vi "tearDown.vi"(8 "error in (no error)":errorcluster, 11 "reference in":refnum<class "Interface Framework Multiple Objects.lvclass">) -> (0 "error out":errorcluster, 3 "reference out":refnum<class "Interface Framework Multiple Objects.lvclass">)   [LabVIEW 2009, in "Interface Framework Multiple Objects.lvclass"]
doc: "tearDown runs after the test method has completed. Use this method to clean up any operations or references that were opened by setUp or the test method. Unit tests should be independent of other unit tests so this VI should ensure that the next test can run in a 'clean' test environment."
uses:
  Interface Framework Multiple Objects.lvclass
  Numeric Test Object/Numeric Test Object.lvclass
  Interface Framework Multiple Objects.lvclass/Interface Framework Multiple Objects.ctl
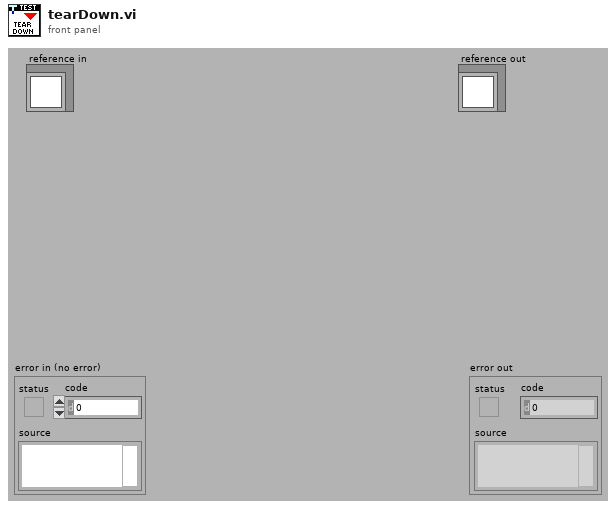
[diagram p1: front panel]
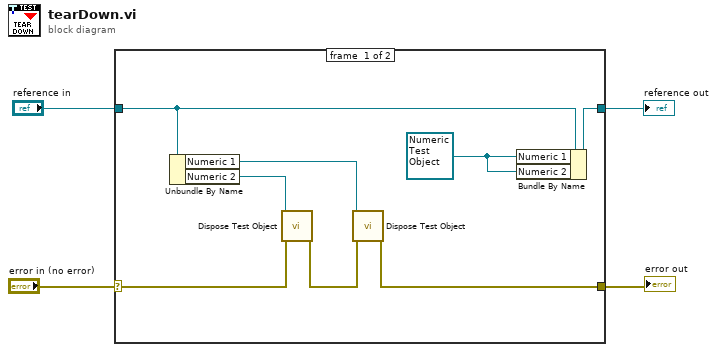
[diagram p0: block diagram]
diagram:
  n1 = case shown="No Error" "error in (no error)" {
    selector: "error in (no error)" -> [w11 w14]
    tunnel: [w9 w14] -> w3
    tunnel: [w6 w13] -> w1
    tunnel: "reference in" -> [w12 w13]
    frame #0 {
      w5 = refnum<class "Numeric Test Object.lvclass"> refnum ("Numeric 1")
      n2 = Unbundle By Name(w12) -> ("Numeric 1"=w7:refnum<class "Numeric Test Object.lvclass">, "Numeric 2"=w8:refnum<class "Numeric Test Object.lvclass">)
      n3 = call "Dispose Test Object.vi"("error in (no error)"=w11, "Numeric"=w8) -> ("error out"=w10:errorcluster)  [unwired: 9 in]
      n4 = call "Dispose Test Object.vi"("error in (no error)"=w10, "Numeric"=w7) -> ("error out"=w9:errorcluster)  [unwired: 9 in]
      n5 = Bundle By Name(cluster=w12, "Numeric 1"=w5, "Numeric 2"=w5) -> (w6:refnum<class "Interface Framework Multiple Objects.lvclass">)
    }
    frame #1 {
    }
  }
  "error out" <- w3
  "reference out" <- w1
